vi "S4P Data Save.vi"(0 "VNA VISA":refnum<visa-resource-name>="TCPIP0::A-N5224A-41544.local::hislip0::INSTR", 1 "VNA Model:":enum16{"E5071C", "N5230A(C)", "N5224A"}(ring)=enum."N5224A", 2 "Sample PN:":string="1111111", 3 "Sample #":i32=1 min=0 step=1, 4 "Pair  Name:":string="TX0", 5 "SampleSN:":string="1111111", 6 "S4P Data Type":enum16{"THRU", "NEXT", "FEXT"}(ring), 8 "Demo Mode":bool, 9 "Channel":string="1") -> (14 "TXT Data Path":path, 15 "S4P File Path":path, 18 "S4P Data Path":path)   [LabVIEW 2011]
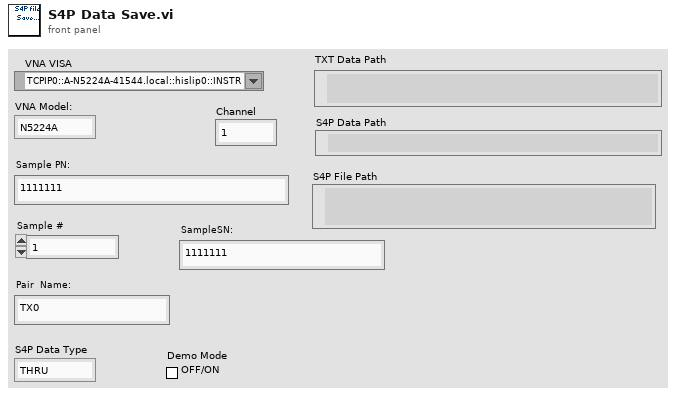
[diagram p1: front panel]
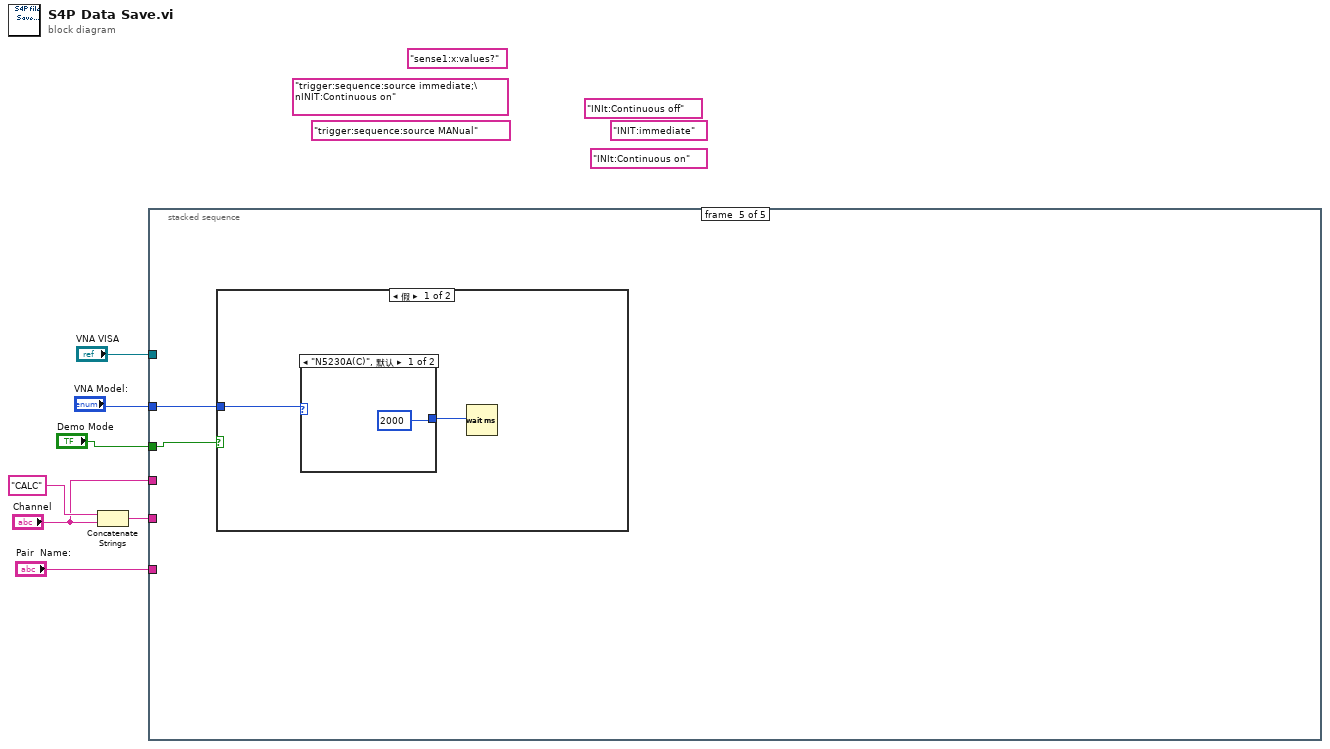
[diagram p0: block diagram]
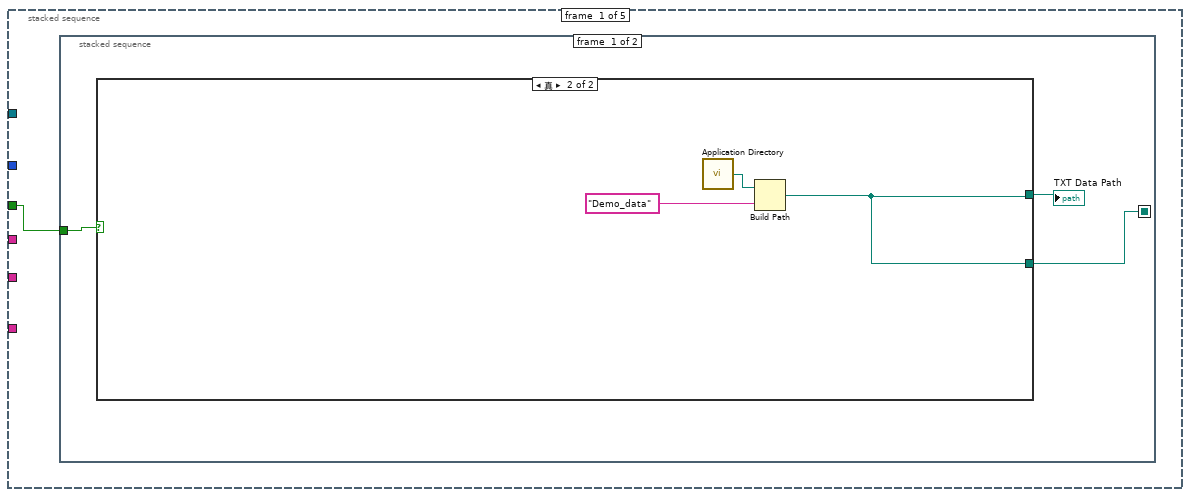
[diagram p2: hidden frame]
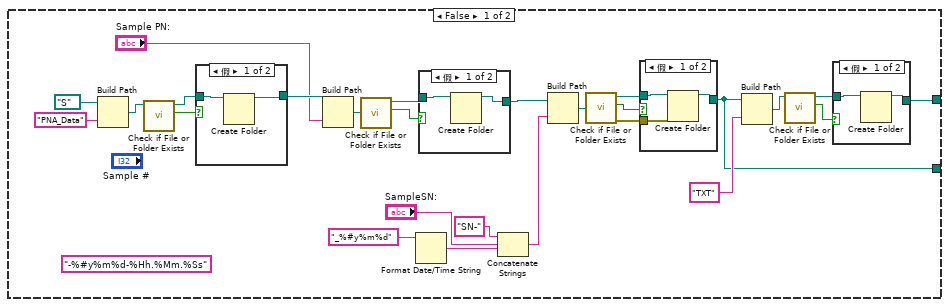
[diagram p3: hidden frame]
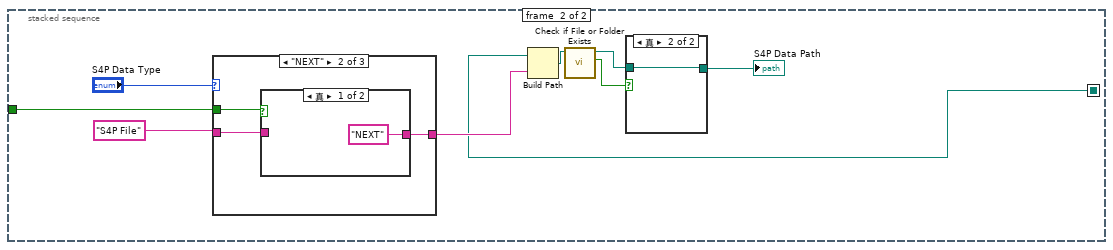
[diagram p8: hidden frame]
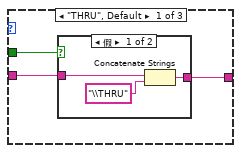
[diagram p9: hidden frame]
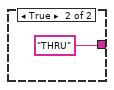
[diagram p10: hidden frame]
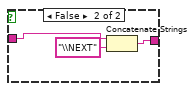
[diagram p11: hidden frame]
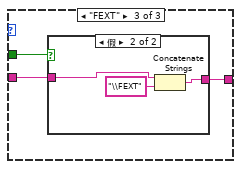
[diagram p12: hidden frame]
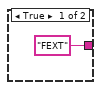
[diagram p13: hidden frame]
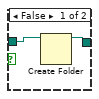
[diagram p14: hidden frame]
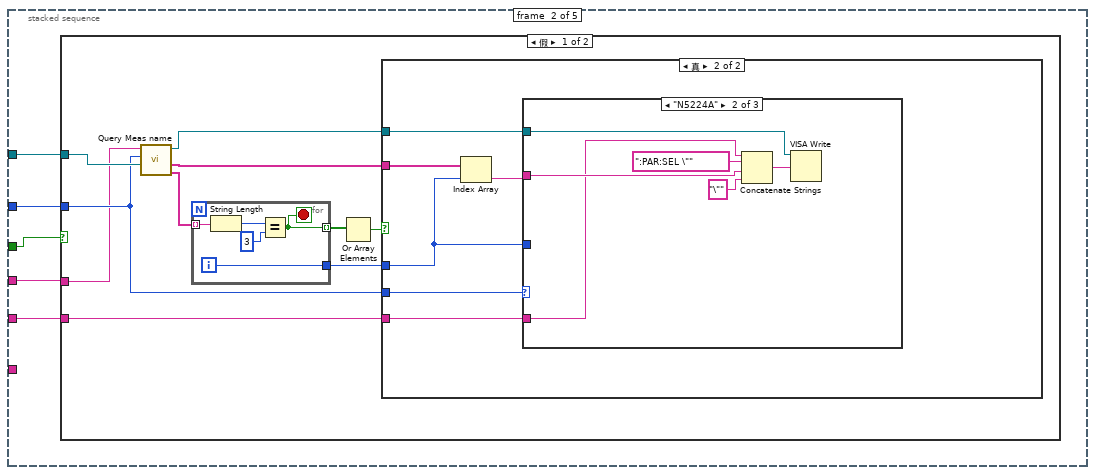
[diagram p15: hidden frame]
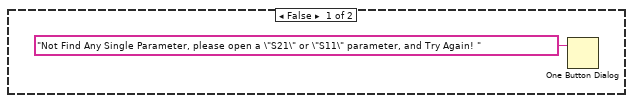
[diagram p16: hidden frame]
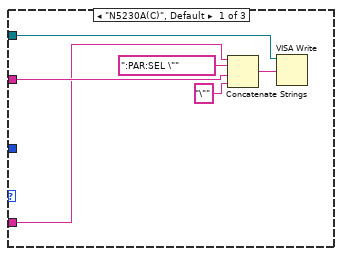
[diagram p17: hidden frame]
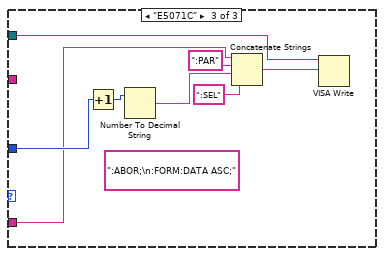
[diagram p18: hidden frame]
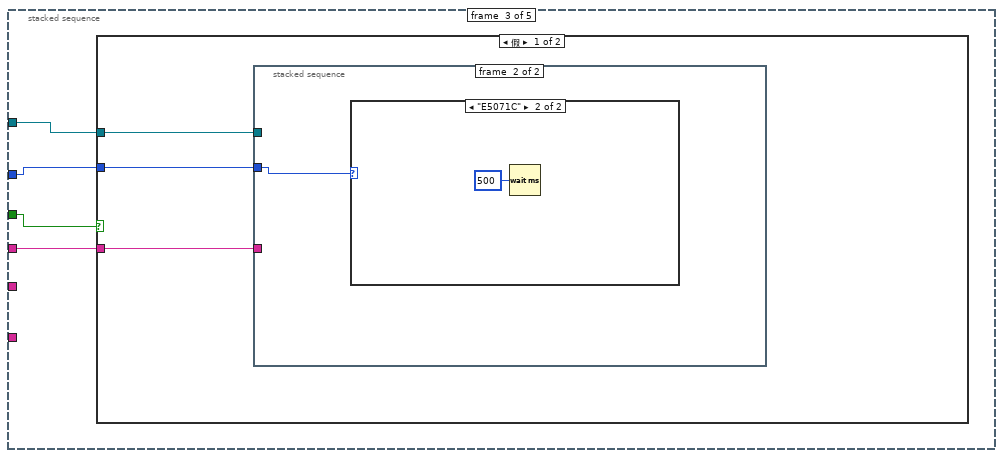
[diagram p20: hidden frame]
diagram:
  (unwired) "INIt:Continuous on" ("write buffer")
  (unwired) "trigger:sequence:source immediate;\nINIT:Continuous on" ("write buffer")
  (unwired) "trigger:sequence:source MANual" ("write buffer")
  (unwired) "INIT:immediate" ("write buffer")
  (unwired) "INIt:Continuous off" ("write buffer")
  (unwired) "sense1:x:values?"
  n1 = Concatenate Strings("CALC" ("字符串"), "Channel") -> (w3:string)
  n2 = stacked-sequence {
    tunnel: "VNA VISA" -> [_ w91 w137 w152 _]
    tunnel: "VNA Model:" -> [_ w90 w136 w151 w190]
    tunnel: "Demo Mode" -> [w8 w89 w135 w150 w189]
    tunnel: w3 -> [_ w87 _ w149 _]
    tunnel: "Channel" -> [_ w88 w134 _ _]
    tunnel: "Pair  Name:" -> [_ _ _ w147 _]
    frame #0 {
      n3 = stacked-sequence {
        seq-local: [w9 _] -> [_ w55]
        tunnel: w8 -> [w10 w54]
        frame #0 {
          n4 = case shown="真" w10 {
            tunnel: [w15 w51] -> w11
            tunnel: [w13 w51] -> w9
            frame False {
              (unwired) "-%#y%m%d-%Hh.%Mm.%Ss" ("time format string (%c)")
              n5 = Build Path(base path=path "S:/" ("基路径"), name or relative path="PNA_Data" ("名称或相对路径")) -> (appended path=w35:path)
              n6 = call <vilib>:"Check if File or Folder Exists.vi"("path"=w35) -> ("file or folder exists?"=w34:bool, "dup path"=w33:path)  [unwired: 8 in, 1 out]
              n7 = case shown="假" w34 {
                tunnel: w33 -> [w49 w50]
                tunnel: [w48 w50] -> w32
                frame False {
                  n8 = Create Folder(path (use dialog)=w49) -> (created path=w48:path)  [unwired: 2 in, 2 out]
                }
                frame True {
                }
              }
              n9 = Build Path(base path=w32, name or relative path="Sample PN:") -> (appended path=w30:path)
              n10 = call <vilib>:"Check if File or Folder Exists.vi"("path"=w30) -> ("file or folder exists?"=w29:bool, "dup path"=w28:path)  [unwired: 8 in, 1 out]
              n11 = Format Date/Time String(time format string (%c)="_%#y%m%d") -> (date/time string=w22:string)  [unwired: 2 in]
              n12 = case shown="假" w29 {
                tunnel: w28 -> [w46 w47]
                tunnel: [w45 w47] -> w27
                frame False {
                  n13 = Create Folder(path (use dialog)=w46) -> (created path=w45:path)  [unwired: 2 in, 2 out]
                }
                frame True {
                }
              }
              n14 = Concatenate Strings("SN-" ("字符串"), "SampleSN:", w22) -> (w21:string)
              n15 = Build Path(base path=w27, name or relative path=w21) -> (appended path=w26:path)
              n16 = call <vilib>:"Check if File or Folder Exists.vi"("path"=w26) -> ("error out"=w12:errorcluster, "file or folder exists?"=w24:bool, "dup path"=w25:path)  [unwired: 8 in]
              n17 = case shown="假" w24 {
                tunnel: w25 -> [w43 w44]
                tunnel: [w42 w44] -> w13
                tunnel: w12 -> [w41 _]
                frame False {
                  n18 = Create Folder(path (use dialog)=w43, error in=w41) -> (created path=w42:path)  [unwired: 1 in, 2 out]
                }
                frame True {
                }
              }
              n19 = Build Path(base path=w13, name or relative path="TXT" ("名称或相对路径")) -> (appended path=w16:path)
              n20 = call <vilib>:"Check if File or Folder Exists.vi"("path"=w16) -> ("file or folder exists?"=w18:bool, "dup path"=w17:path)  [unwired: 8 in, 1 out]
              n21 = case shown="假" w18 {
                tunnel: w17 -> [w39 w40]
                tunnel: [w38 w40] -> w15
                frame False {
                  n22 = Create Folder(path (use dialog)=w39) -> (created path=w38:path)  [unwired: 2 in, 2 out]
                }
                frame True {
                }
              }
            }
            frame True {
              n23 = call <vilib>:"Application Directory.vi"() -> ("Application Directory"=w53:path)
              n24 = Build Path(base path=w53, name or relative path="Demo_data" ("名称或相对路径")) -> (appended path=w51:path)
            }
          }
          "TXT Data Path" <- w11
        }
        frame #1 {
          n25 = case shown="\"NEXT\"" "S4P Data Type" {
            tunnel: "S4P File" ("名称或相对路径") -> [w65 w72 w79]
            tunnel: [w64 w71 w78] -> w56
            tunnel: w54 -> [w63 w70 w77]
            frame "THRU", Default {
              n26 = case shown="假" w63 {
                tunnel: w65 -> [w68 _]
                tunnel: [w66 "THRU" ("字符串")] -> w64
                frame False {
                  n27 = Concatenate Strings(w68, "\\THRU" ("字符串")) -> (w66:string)
                }
                frame True {
                }
              }
            }
            frame "NEXT" {
              n28 = case shown="真" w70 {
                tunnel: w72 -> [_ w76]
                tunnel: ["NEXT" ("字符串") w74] -> w71
                frame True {
                }
                frame False {
                  n29 = Concatenate Strings(w76, "\\NEXT" ("字符串")) -> (w74:string)
                }
              }
            }
            frame "FEXT" {
              n30 = case shown="假" w77 {
                tunnel: w79 -> [_ w83]
                tunnel: ["FEXT" ("字符串") w81] -> w78
                frame True {
                }
                frame False {
                  n31 = Concatenate Strings(w83, "\\FEXT" ("字符串")) -> (w81:string)
                }
              }
            }
          }
          n32 = Build Path(base path=w55, name or relative path=w56) -> (appended path=w62:path)
          n33 = call <vilib>:"Check if File or Folder Exists.vi"("path"=w62) -> ("file or folder exists?"=w61:bool, "dup path"=w60:path)  [unwired: 8 in, 1 out]
          n34 = case shown="真" w61 {
            tunnel: w60 -> [w85 w86]
            tunnel: [w84 w86] -> w59
            frame False {
              n35 = Create Folder(path (use dialog)=w85) -> (created path=w84:path)  [unwired: 2 in, 2 out]
            }
            frame True {
            }
          }
          "S4P Data Path" <- w59
        }
      }
    }
    frame #1 {
      n36 = case shown="假" w89 {
        tunnel: w91 -> [w101 _]
        tunnel: w90 -> [w98 _]
        tunnel: w88 -> [w97 _]
        tunnel: w87 -> [w96 _]
        frame False {
          n37 = call "Query Meas name.vi"("VISA resource name"=w101, "VNA Model"=w98, "Channel"=w97) -> ("Parameter item"=w95:string[], "Name list"=w100:string[], "Dup VISA resource name"=w99:refnum<visa-resource-name>)  [unwired: 4 in]
          n38 = for {
            tunnel: w95 -> [w133] mode=indexing
            tunnel: [w130] -> w93 mode=indexing
            tunnel: [w129] -> w94
            i -> [w129]
            stop <- w130 stop-if-true
            n39 = String Length(string=w133) -> (length=w132:i32)
            n40 = Equal?(x=w132, y=3) -> (x = y?=w130:bool)
          }
          n41 = Or Array Elements(Boolean array=w93) -> (logical OR=w92:bool)
          n42 = case shown="真" w92 {
            tunnel: w100 -> [_ w108]
            tunnel: w99 -> [_ w107]
            tunnel: w98 -> [_ w106]
            tunnel: w96 -> [_ w104]
            tunnel: w94 -> [_ w103]
            frame False {
              n43 = One Button Dialog(message="Not Find Any Single Parameter, please open a \"S21\" or \"S11\" parameter, and Try Again! " ("消息")) -> ()  [unwired: 1 in, 1 out]
            }
            frame True {
              n44 = Index Array(array=w108, index=w103) -> (element=w105:string)
              n45 = case shown="\"N5224A\"" w106 {
                tunnel: w107 -> [w111 w117 w125]
                tunnel: w105 -> [w110 w116 _]
                tunnel: w103 -> [_ _ w123]
                tunnel: w104 -> [w109 w115 w121]
                frame "N5230A(C)", Default {
                  n46 = Concatenate Strings(w109, ":PAR:SEL \"", w110, "\"" ("string")) -> (w112:string)
                  n47 = VISA Write(VISA resource name=w111, write buffer=w112) -> ()  [unwired: 1 in, 3 out]
                }
                frame "N5224A" {
                  n48 = Concatenate Strings(w115, ":PAR:SEL \"", w116, "\"" ("string")) -> (w118:string)
                  n49 = VISA Write(VISA resource name=w117, write buffer=w118) -> ()  [unwired: 1 in, 3 out]
                }
                frame "E5071C" {
                  (unwired) ":ABOR;\n:FORM:DATA ASC;"
                  n50 = Increment(x=w123) -> (x+1=w124:i32)
                  n51 = Number To Decimal String(number=w124) -> (decimal integer string=w122:string)  [unwired: 1 in]
                  n52 = Concatenate Strings(w121, ":PAR" ("string"), w122, ":SEL" ("string")) -> (w128:string)
                  n53 = VISA Write(VISA resource name=w125, write buffer=w128) -> ()  [unwired: 1 in, 3 out]
                }
              }
            }
          }
        }
        frame True {
        }
      }
    }
    frame #2 {
      n54 = case shown="假" w135 {
        tunnel: w137 -> [w140 _]
        tunnel: w136 -> [w139 _]
        tunnel: w134 -> [w138 _]
        frame False {
          n55 = stacked-sequence {
            tunnel: w140 -> [w142 _]
            tunnel: w139 -> [w143 w144]
            tunnel: w138 -> [w141 _]
            frame #0 {
              n56 = call "Single Triger.vi"("Channel"=w141, "VNA Model:"=w143, "VISA"=w142) -> ()  [unwired: 9 in]
            }
            frame #1 {
              n57 = case shown="\"E5071C\"" w144 {
                frame "N5230A(C)", Default {
                  n58 = Wait (ms)(milliseconds to wait=u32 500 ("等待时间（毫秒）")) -> ()  [unwired: 1 out]
                }
                frame "E5071C" {
                  n59 = Wait (ms)(milliseconds to wait=u32 500 ("等待时间（毫秒）")) -> ()  [unwired: 1 out]
                }
              }
            }
          }
        }
        frame True {
        }
      }
    }
    frame #3 {
      n60 = case shown="假" w150 {
        tunnel: w152 -> [w166 _]
        tunnel: w151 -> [w165 _]
        tunnel: w149 -> [w164 _]
        tunnel: [w156 w184] -> w148
        tunnel: w147 -> [w155 w185]
        frame False {
          (unwired) "\\\\172.20.61.12\\\\1111111\\Sample_#1_150330\\S4P File\\THRU" ("字符串")
          # "\\\\172.20.61.12\\PNA_Data"
          n61 = local read "S4P Data Path"() -> (w153:path)
          n62 = Concatenate Strings(w155, ".s4p" ("字符串")) -> (w160:string)
          n63 = Build Path(base path=w153, name or relative path=w160) -> (appended path=w156:path)
          n64 = Path To String(path=w156) -> (string=w154:string)
          n65 = Concatenate Strings(w154, " '" ("字符串")) -> (w157:string)
          n66 = case shown="\"E5071C\"" w165 {
            tunnel: ["MMEM:STOR:TRAC:FORM:SNP RI" ("写入缓冲区") "MMEM:STOR:TRAC:FORM:SNP RI" ("写入缓冲区") ":MMEM:STOR:SNP:FORM RI" ("写入缓冲区")] -> w163
            tunnel: [w169 w174 w182] -> w161
            tunnel: w157 -> [w170 w175 _]
            tunnel: w164 -> [w167 w172 _]
            tunnel: w154 -> [_ _ w178]
            frame "N5230A(C)", Default {
              (unwired) "MMEM:STOR:TRAC:FORM:SNP DB" ("写入缓冲区")
              (unwired) "MMEM:STOR:TRAC:FORM:SNP MA" ("写入缓冲区")
              n67 = Concatenate Strings(w167, ":DATA:SNP:PORTs:Save '1,2,3,4', '" ("写入缓冲区"), w170) -> (w169:string)
            }
            frame "N5224A" {
              (unwired) "MMEM:STOR:TRAC:FORM:SNP DB" ("写入缓冲区")
              (unwired) "MMEM:STOR:TRAC:FORM:SNP MA" ("写入缓冲区")
              n68 = Concatenate Strings(w172, ":DATA:SNP:PORTs:Save '1,2,3,4', '" ("写入缓冲区"), w175) -> (w174:string)
            }
            frame "E5071C" {
              n69 = Concatenate Strings(":MMEM:STOR:SNP:TYPE:S4P 1,2,3,4" ("write buffer"), ";" ("字符串"), ":MMEM:STOR:SNP \"" ("写入缓冲区"), w178, "\"" ("字符串")) -> (w182:string)
            }
          }
          n70 = VISA Write(VISA resource name=w166, write buffer=w163) -> (VISA resource name out=w162:refnum<visa-resource-name>)  [unwired: 1 in, 2 out]
          n71 = VISA Write(VISA resource name=w162, write buffer=w161) -> ()  [unwired: 1 in, 3 out]
        }
        frame True {
          n72 = local read "S4P Data Path"() -> (w188:path)
          n73 = Concatenate Strings(w185, ".s4p" ("字符串")) -> (w187:string)
          n74 = Build Path(base path=w188, name or relative path=w187) -> (appended path=w184:path)
        }
      }
      "S4P File Path" <- w148
    }
    frame #4 {
      n75 = case shown="假" w189 {
        tunnel: w190 -> [w192 _]
        frame False {
          n76 = case shown="\"N5230A(C)\", 默认" w192 {
            tunnel: [u32 2000 ("等待时间（毫秒）") u32 2500 ("等待时间（毫秒）")] -> w191
            frame "N5230A(C)", Default {
            }
            frame "E5071C" {
            }
          }
          n77 = Wait (ms)(milliseconds to wait=w191) -> ()  [unwired: 1 out]
        }
        frame True {
        }
      }
    }
  }
